vi "Variant to Value Objects.vi"(5 "Group Index":i32, 6 "types in":T1[](array[typedef]), 7 "Name Root":string, 8 "error in (no error)":errorcluster, 9 "Value Objects IN":refnum<class "Abs_Value.lvclass">[](array[class]), 10 "Variant":variant, 11 "bt_Blackboard in":refnum<class "Blackboard.lvclass">) -> (0 "error out":errorcluster, 1 "Value Objects OUT":refnum<class "Abs_Value.lvclass">[](array[class]), 3 "bt_Blackboard out":refnum<class "Blackboard.lvclass">, 4 "types out":T1[](array[typedef]))   [LabVIEW 2021, in "BT.lvlib" / "bt_WaitOn_Synch_WithValues.lvclass"]
uses:
  bt_WaitOn_Synch_WithValues.lvclass
  <vilib>/Utility/Data Type/Type Definitions/Data Type.ctl
  Blackboard/Blackboard.lvclass
  <vilib>/TSA/Abstract Data Classes/Abs_Types/Value/Abs_Value.lvclass
  Blackboard/Blackboard.lvclass/Blackboard.ctl
  <vilib>/TSA/Omni-Bus/Local Bus/Support/DBL/Local Bus_DBL.lvclass
  C:/Program Files (x86)/National Instruments/LabVIEW 2021/vi.lib/TSA/Abstract Data Classes/Abs_Types/Value/Abs_Value.lvclass
  <vilib>/TSA/Omni-Bus/Local Bus/Support/SGL/Local Bus_SGL.lvclass
  <vilib>/TSA/Omni-Bus/Local Bus/Support/EXT/Local Bus_EXT.lvclass
  <vilib>/TSA/Omni-Bus/Local Bus/Support/Bool/Local Bus_Boolean.lvclass
  <vilib>/TSA/Omni-Bus/Local Bus/Support/STR/Local Bus_String.lvclass
  <vilib>/TSA/Omni-Bus/Local Bus/Support/Variant/Local Bus_Variant.lvclass
  <vilib>/TSA/Omni-Bus/Local Bus/Support/WFM/Local Bus_Waveform.lvclass
  <vilib>/TSA/Omni-Bus/Local Bus/Support/Time/Local Bus_Time.lvclass
  <vilib>/TSA/Omni-Bus/Local Bus/Support/U8/Local Bus_U8.lvclass
  <vilib>/TSA/Omni-Bus/Local Bus/Support/U16/Local Bus_U16.lvclass
  <vilib>/TSA/Omni-Bus/Local Bus/Support/U32/Local Bus_U32.lvclass
  <vilib>/TSA/Omni-Bus/Local Bus/Support/U64/Local Bus_U64.lvclass
  <vilib>/TSA/Omni-Bus/Local Bus/Support/I8/Local Bus_I8.lvclass
  <vilib>/TSA/Omni-Bus/Local Bus/Support/I16/Local Bus_I16.lvclass
  <vilib>/TSA/Omni-Bus/Local Bus/Support/I32/Local Bus_I32.lvclass
  <vilib>/TSA/Omni-Bus/Local Bus/Support/I64/Local Bus_I64.lvclass
  <vilib>/TSA/Omni-Bus/Local Bus/Support/CSGL/Local Bus_CSGL.lvclass
  <vilib>/TSA/Omni-Bus/Local Bus/Support/CDBL/Local Bus_CDBL.lvclass
  <vilib>/TSA/Omni-Bus/Local Bus/Support/CEXT/Local Bus_CEXT.lvclass
  <vilib>/Utility/error.llb/Error Cluster From Error Code.vi
  <vilib>/ErrorRing/Error Ring.xnode
  <vilib>/TSA/Omni-Bus/Local Bus/Support/Type/Local Bus_Type.lvclass
  <vilib>/TSA/Abstract Data Classes/Abs_Types/Type/Abs_Type.lvclass
  <vilib>/Utility/Data Type/NI_Data Type.lvlib
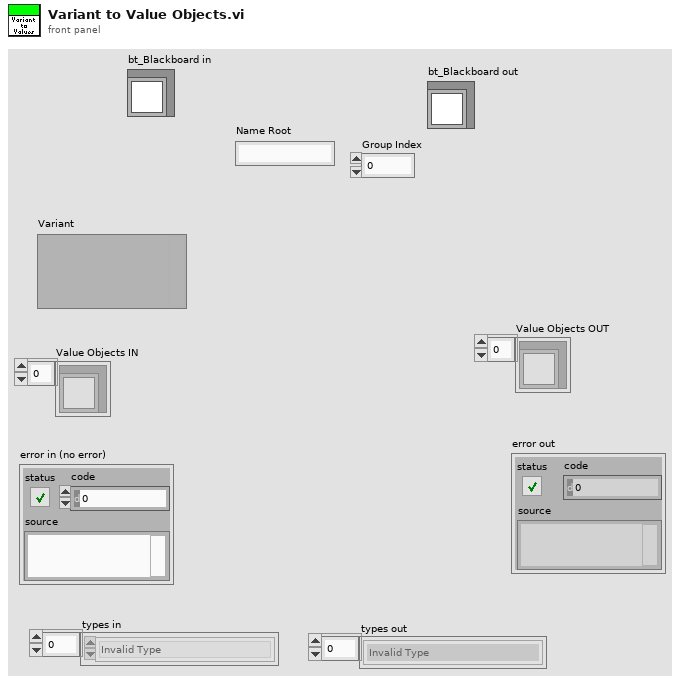
[diagram p1: front panel]
types:
  T1 = typedef "NI_Data Type.lvlib/Data Type.ctl" = enum8{"Invalid Type", "Void", "I8", "I16", "I32", "I64", "U8", "U16", "U32", "U64", "Single Float", "Double Float", "Extended Float", "Single Complex", "Double Complex", "Extended Complex", "Enum U8", "Enum U16", "Enum U32", "Enum U64", "Single Float With Unit", "Double Float With Unit", "Extended Float With Unit", "Single Complex with Unit", "Double Complex with Unit", "Extended Complex with Unit", "Boolean", "String", "Path", "Picture", "Tag", "Array", "Cluster", "Variant", "LV Variant", "Waveform", "Timestamp", "Digital Waveform", "Digital Data", "ExpressData", "Refnum", "External Data", "VI", "Poly VI", "LabVIEW Class Instance", "Fixed Point", "Set Collection", "Map Collection"}
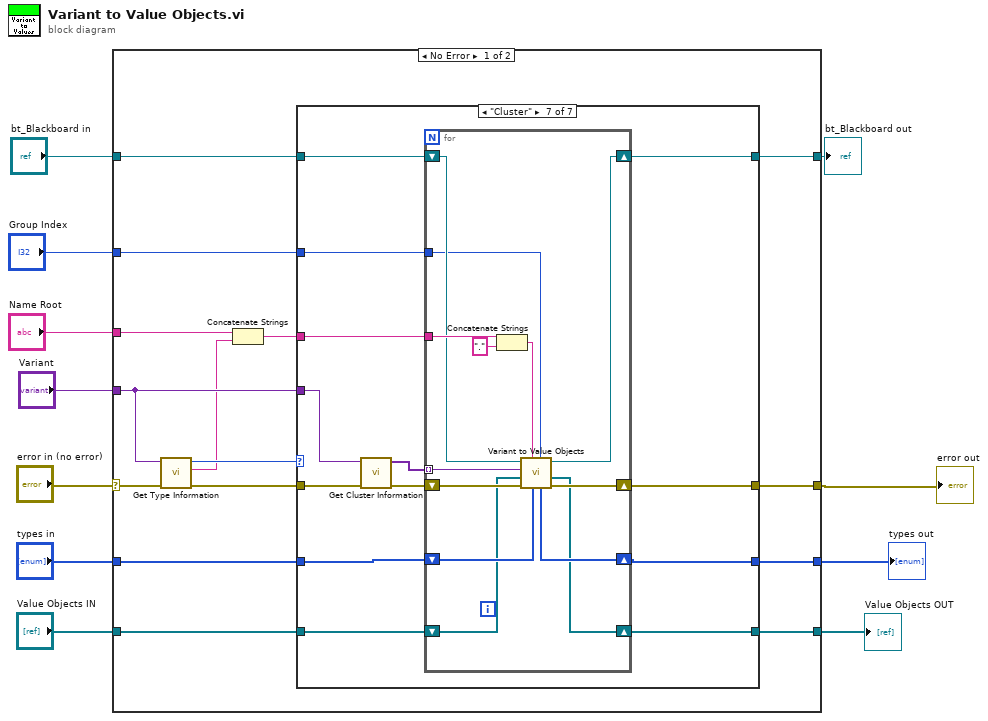
[diagram p0: block diagram]
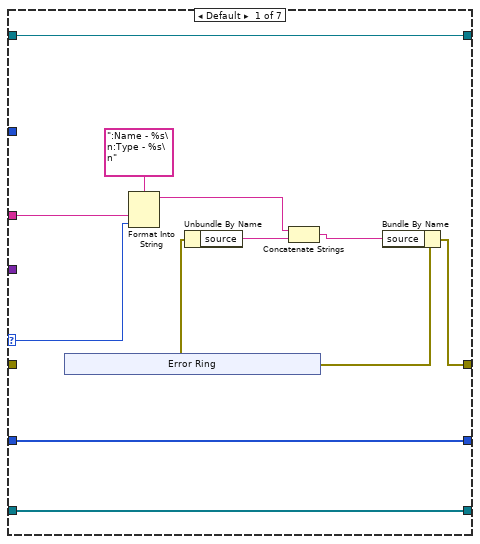
[diagram p2: hidden frame]
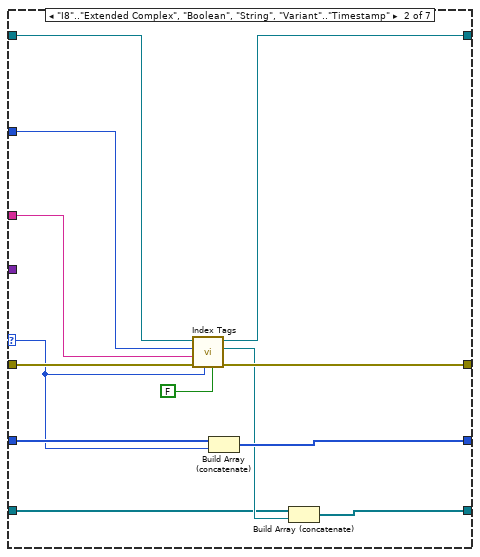
[diagram p3: hidden frame]
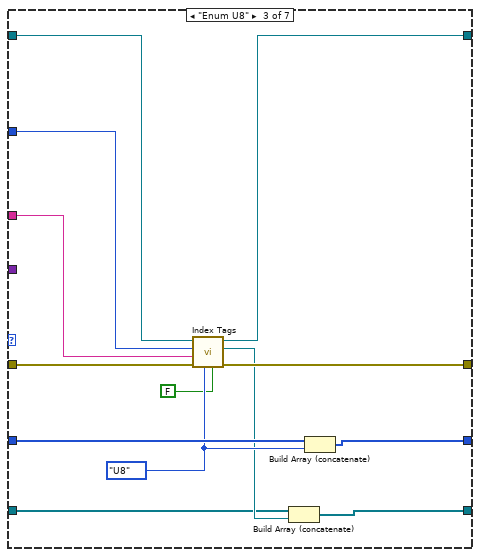
[diagram p4: hidden frame]
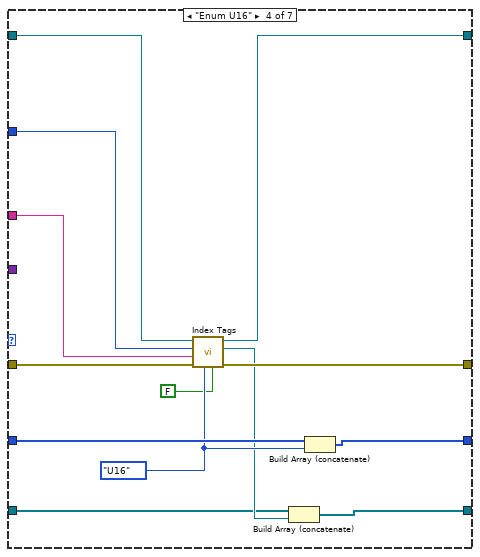
[diagram p5: hidden frame]
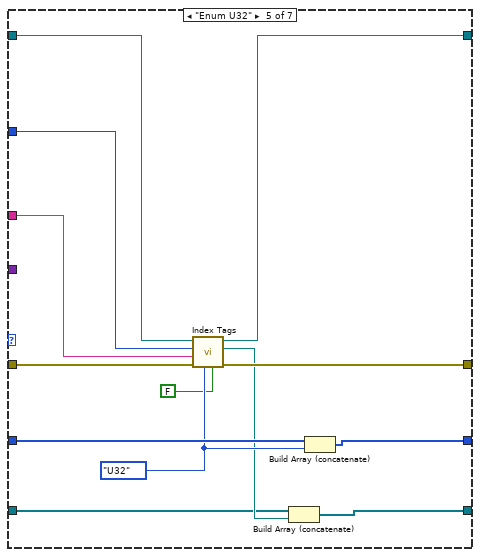
[diagram p6: hidden frame]
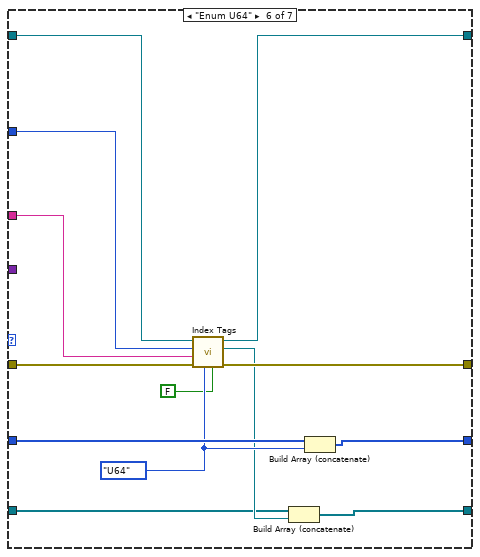
[diagram p7: hidden frame]
diagram:
  n1 = case shown="No Error" "error in (no error)" {
    selector: "error in (no error)" -> [w26 w135]
    tunnel: "Variant" -> [w23 _]
    tunnel: "Name Root" -> [w20 _]
    tunnel: "types in" -> [w19 w134]
    tunnel: [w18 w134] -> w7
    tunnel: [w17 w135] -> w6
    tunnel: "bt_Blackboard in" -> [w16 w136]
    tunnel: "Group Index" -> [w15 _]
    tunnel: [w14 w136] -> w3
    tunnel: [w13 w133] -> w2
    tunnel: "Value Objects IN" -> [w12 w133]
    frame No Error {
      n2 = call <vilib>:"Get Type Information.vi"("error in (no error)"=w26, "variant"=w23) -> ("error out"=w24:errorcluster, "name"=w21:string, "type"=w25:T1)  [unwired: 5 in, 2 out]
      n3 = Concatenate Strings(w20, w21) -> (w22:string)
      n4 = case shown="\"Cluster\"" w25 {
        selector: w25 -> [w27 w46 _ _ _ _ _]
        tunnel: w24 -> [_ w52 w65 w78 w91 w104 w119]
        tunnel: w23 -> [_ _ _ _ _ _ w118]
        tunnel: [w34 w51 w64 w77 w90 w103 w115] -> w17
        tunnel: w22 -> [w28 w49 w62 w75 w88 w101 w114]
        tunnel: w19 -> [w37 w54 w67 w80 w93 w106 w113]
        tunnel: [w37 w53 w66 w79 w92 w105 w112] -> w18
        tunnel: w16 -> [w36 w50 w63 w76 w89 w102 w111]
        tunnel: w15 -> [_ w48 w61 w74 w87 w100 w109]
        tunnel: [w36 w47 w60 w73 w86 w99 w110] -> w14
        tunnel: [w35 w43 w56 w69 w82 w95 w107] -> w13
        tunnel: w12 -> [w35 w42 w55 w68 w81 w94 w108]
        frame Default {
          n5 = xnode "Error Ring"() -> ("error out"=w33:errorcluster)
          n6 = Format Into String(format string=":Name - %s\n:Type - %s\n", w28, w27) -> (resulting string=w29:string)  [unwired: 2 in, 1 out]
          n7 = Unbundle By Name(w33) -> ("source"=w32:string)
          n8 = Concatenate Strings(w29, w32) -> (w31:string)
          n9 = Bundle By Name(cluster=w33, "source"=w31) -> (w34:errorcluster)
        }
        frame "I8".."Extended Complex", "Boolean", "String", "Variant".."Timestamp" {
          n10 = call "Index Tags.vi"("Don't Create"=FALSE, "Tag Type"=w46, "error in (no error)"=w52, "Tag"=w49, "Group Index"=w48, "bt_Blackboard in"=w50) -> ("error out"=w51:errorcluster, "Value"=w44:refnum<class "Abs_Value.lvclass">, "bt_Blackboard out"=w47:refnum<class "Blackboard.lvclass">)  [unwired: 2 in, 1 out]
          n11 = Build Array (concatenate)(w54, w46) -> (w53:T1[])
          n12 = Build Array (concatenate)(w42, w44) -> (w43:refnum<class "Abs_Value.lvclass">[])
        }
        frame "Enum U8" {
          w59 = Data_Type."U8" ("Tag Type")
          n13 = call "Index Tags.vi"("Don't Create"=FALSE, "Tag Type"=w59, "error in (no error)"=w65, "Tag"=w62, "Group Index"=w61, "bt_Blackboard in"=w63) -> ("error out"=w64:errorcluster, "Value"=w57:refnum<class "Abs_Value.lvclass">, "bt_Blackboard out"=w60:refnum<class "Blackboard.lvclass">)  [unwired: 2 in, 1 out]
          n14 = Build Array (concatenate)(w55, w57) -> (w56:refnum<class "Abs_Value.lvclass">[])
          n15 = Build Array (concatenate)(w67, w59) -> (w66:T1[])
        }
        frame "Enum U16" {
          w72 = Data_Type."U16" ("Tag Type")
          n16 = call "Index Tags.vi"("Don't Create"=FALSE, "Tag Type"=w72, "error in (no error)"=w78, "Tag"=w75, "Group Index"=w74, "bt_Blackboard in"=w76) -> ("error out"=w77:errorcluster, "Value"=w70:refnum<class "Abs_Value.lvclass">, "bt_Blackboard out"=w73:refnum<class "Blackboard.lvclass">)  [unwired: 2 in, 1 out]
          n17 = Build Array (concatenate)(w68, w70) -> (w69:refnum<class "Abs_Value.lvclass">[])
          n18 = Build Array (concatenate)(w80, w72) -> (w79:T1[])
        }
        frame "Enum U32" {
          w85 = Data_Type."U32" ("Tag Type")
          n19 = call "Index Tags.vi"("Don't Create"=FALSE, "Tag Type"=w85, "error in (no error)"=w91, "Tag"=w88, "Group Index"=w87, "bt_Blackboard in"=w89) -> ("error out"=w90:errorcluster, "Value"=w83:refnum<class "Abs_Value.lvclass">, "bt_Blackboard out"=w86:refnum<class "Blackboard.lvclass">)  [unwired: 2 in, 1 out]
          n20 = Build Array (concatenate)(w81, w83) -> (w82:refnum<class "Abs_Value.lvclass">[])
          n21 = Build Array (concatenate)(w93, w85) -> (w92:T1[])
        }
        frame "Enum U64" {
          w98 = Data_Type."U64" ("Tag Type")
          n22 = call "Index Tags.vi"("Don't Create"=FALSE, "Tag Type"=w98, "error in (no error)"=w104, "Tag"=w101, "Group Index"=w100, "bt_Blackboard in"=w102) -> ("error out"=w103:errorcluster, "Value"=w96:refnum<class "Abs_Value.lvclass">, "bt_Blackboard out"=w99:refnum<class "Blackboard.lvclass">)  [unwired: 2 in, 1 out]
          n23 = Build Array (concatenate)(w94, w96) -> (w95:refnum<class "Abs_Value.lvclass">[])
          n24 = Build Array (concatenate)(w106, w98) -> (w105:T1[])
        }
        frame "Cluster" {
          n25 = call <vilib>:"Get Cluster Information.vi"("error in (no error)"=w119, "variant"=w118) -> ("error out"=w117:errorcluster, "cluster elements"=w116:variant[])  [unwired: 8 in]
          n26 = for {
            tunnel: w116 -> [w125] mode=indexing
            shift-right: [w131] -> w115
            shift-left: w117 -> [w132]
            tunnel: w114 -> [w130]
            shift-right: [w126] -> w112
            shift-left: w113 -> [w127]
            shift-right: [w123] -> w110
            shift-left: w111 -> [w124]
            tunnel: w109 -> [w122]
            shift-right: [w120] -> w107
            shift-left: w108 -> [w121]
            n27 = Concatenate Strings(w130, "." ("string")) -> (w128:string)
            n28 = call "Variant to Value Objects.vi"("Group Index"=w122, "types in"=w127, "Name Root"=w128, "error in (no error)"=w132, "Value Objects IN"=w121, "Variant"=w125, "bt_Blackboard in"=w124) -> ("error out"=w131:errorcluster, "Value Objects OUT"=w120:refnum<class "Abs_Value.lvclass">[], "bt_Blackboard out"=w123:refnum<class "Blackboard.lvclass">, "types out"=w126:T1[])  [unwired: 1 in]
          }
        }
      }
    }
    frame Error {
    }
  }
  "error out" <- w6
  "types out" <- w7
  "bt_Blackboard out" <- w3
  "Value Objects OUT" <- w2
